vi "CODCr流程质控自动启动.vi"(0 "参数":T1={"是否启用仪器"=FALSE, "CODCr"={"启动测量模式"={"测量模式"=enum."水样测量"}, "确定按钮"=TRUE}, "启动模块"={"氨氮"=FALSE, "总磷"=FALSE, "总氮"=FALSE, "COD"=FALSE}, "常规启动"=FALSE, "直接启动"=FALSE}, 1 "CODCr量程切换":enum32{"H", "L", "AUTO"}(ring)=enum."AUTO" caption="CODMn量程切换") -> ()   [LabVIEW 2016, in "质控单元.lvlib"]
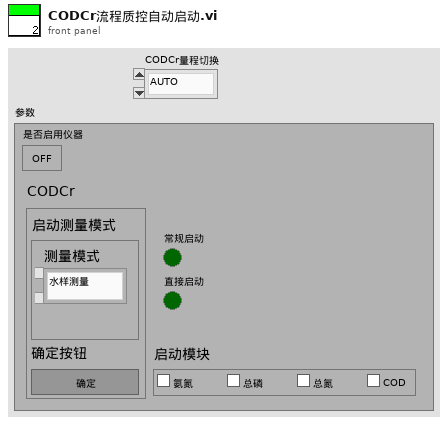
[diagram p1: front panel]
types:
  T1 = cluster{"是否启用仪器":bool, "CODCr":cluster{"启动测量模式":cluster{"测量模式":enum16{"水样测量", "标样核查", "加标回收", "平行样", "校零", "校标"}}, "确定按钮":bool}, "启动模块":cluster{"氨氮":bool, "总磷":bool, "总氮":bool, "COD":bool}, "常规启动":bool, "直接启动":bool}
  T2 = cluster{"R0":i16, "R1":i16, "R2":i16, "R3":i16, "R4":i16, "R5":i16, "R6":i16, "R7":i16, "R8":i16, "R9":i16, "R10":i16, "R11":i16, "R12":i16, "R13":i16, "R14":i16, "R15":i16, "R16":i16, "R17":i16, "R18":i16, "R19":i16, "R20":i16, "R21":i16, "R22":i16, "R23":i16, "R24":i16, "R25":i16, "R26":i16, "R27":i16, "R28":i16, "R29":i16, "R30":i16, "R31":i16, "R32":i16, "R33":i16, "R34":i16, "R35":i16, "R36":i16, "R37":i16, "R38":i16, "R39":i16, "R40":i16, "R41":i16, "R42":i16, "R43":i16, "R44":i16, "R45":i16, "R46":i16, "R47":i16, "R48":i16, "R49":i16, "R50":i16, "R51":i16, "R52":i16, "R53":i16, "R54":i16, "R55":i16, "R56":i16}
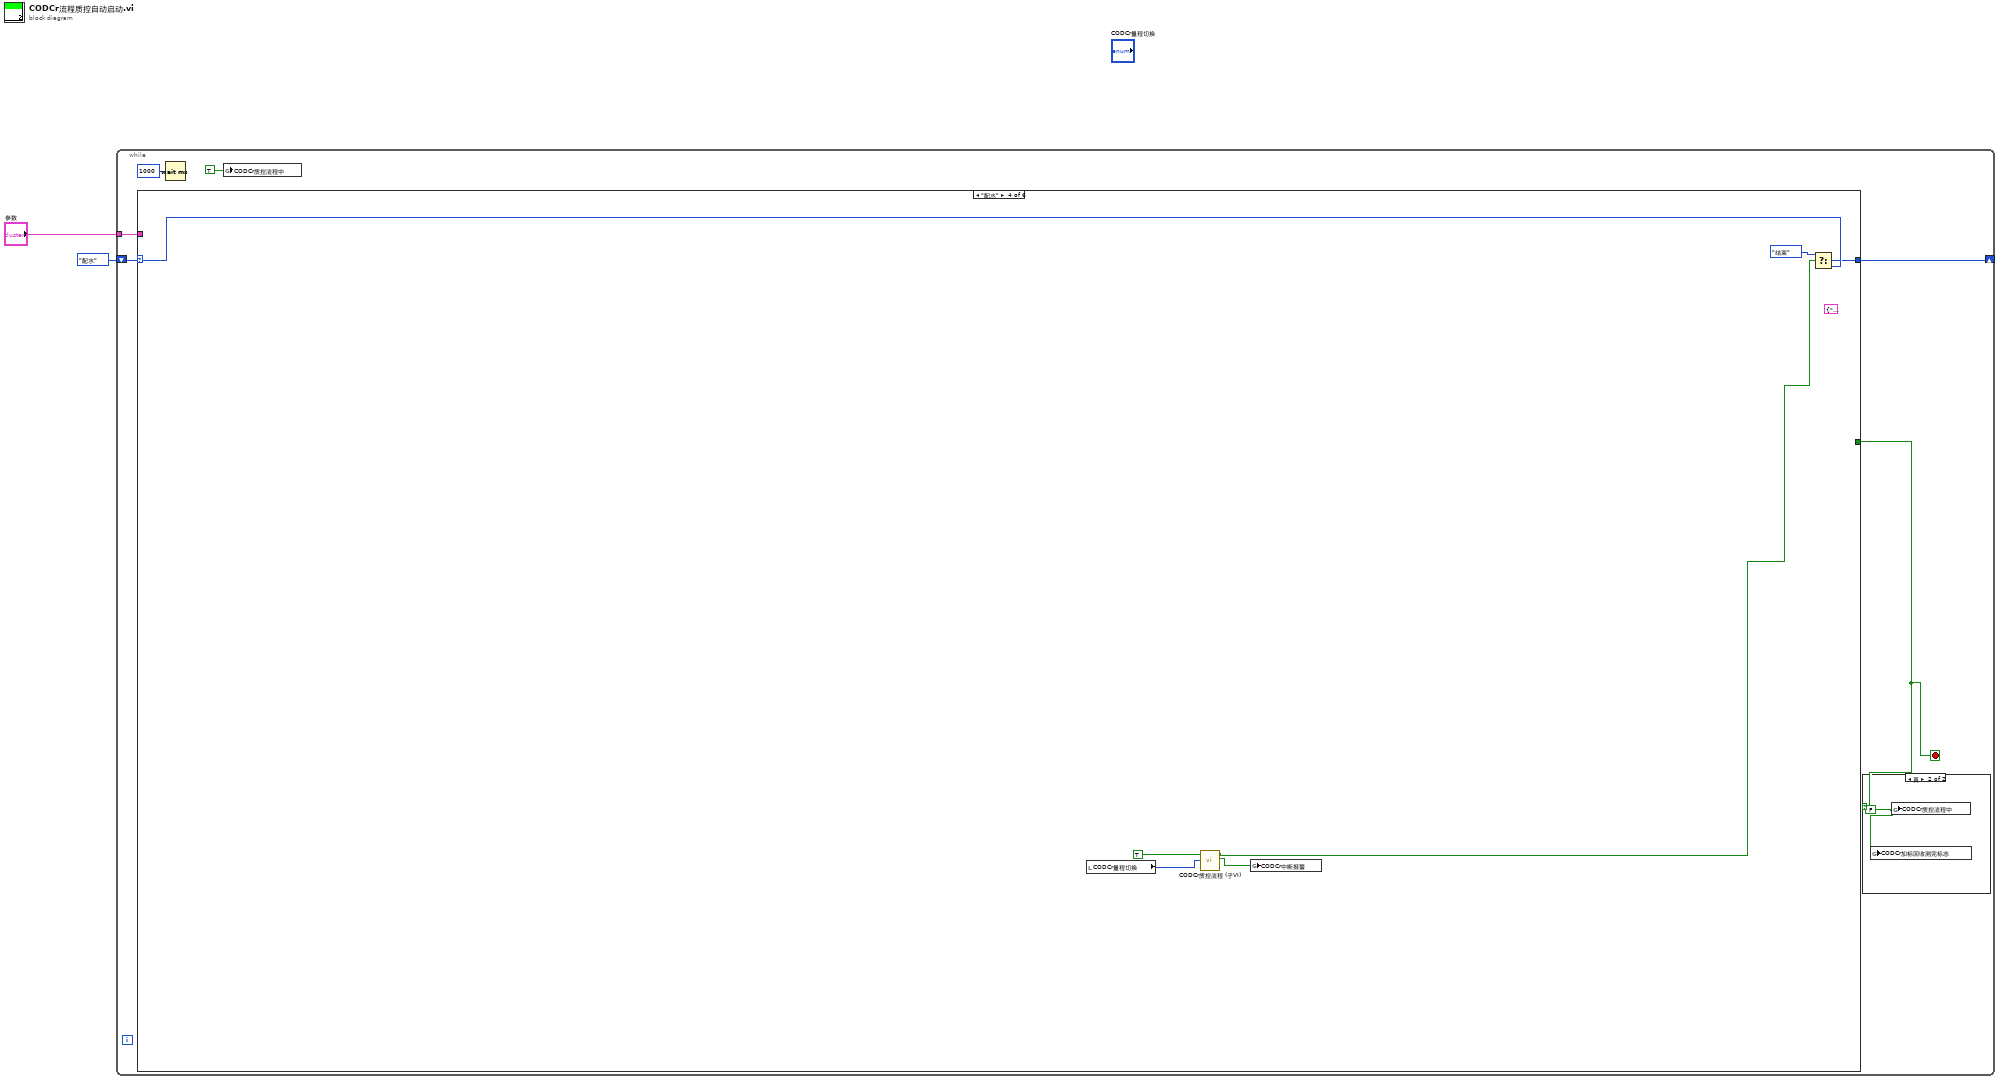
[diagram p0: block diagram]
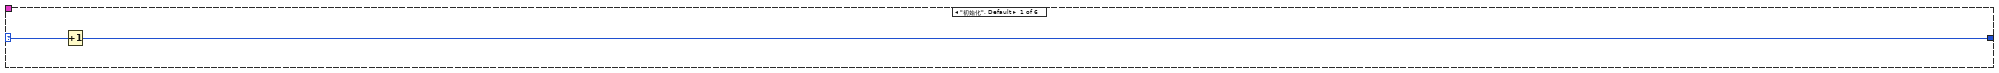
[diagram p3: hidden frame]
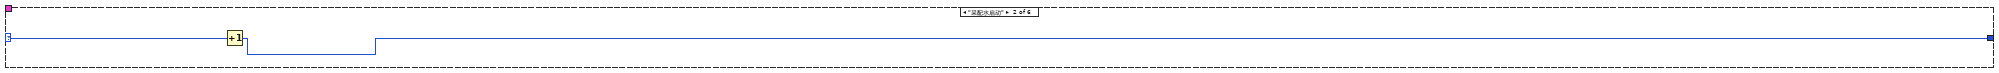
[diagram p4: hidden frame]
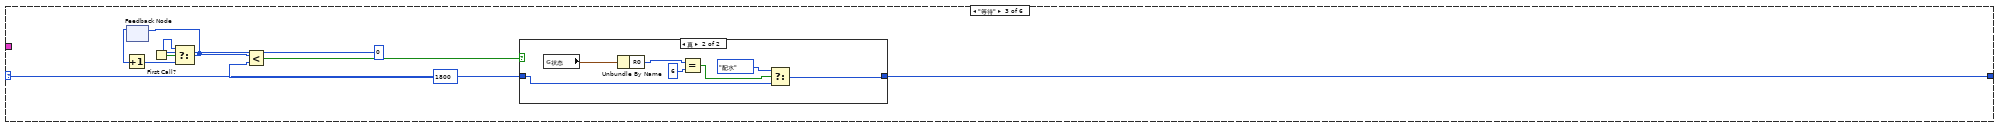
[diagram p5: hidden frame]
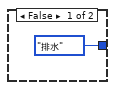
[diagram p6: hidden frame]
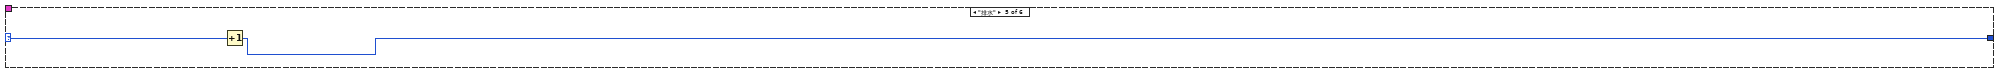
[diagram p7: hidden frame]
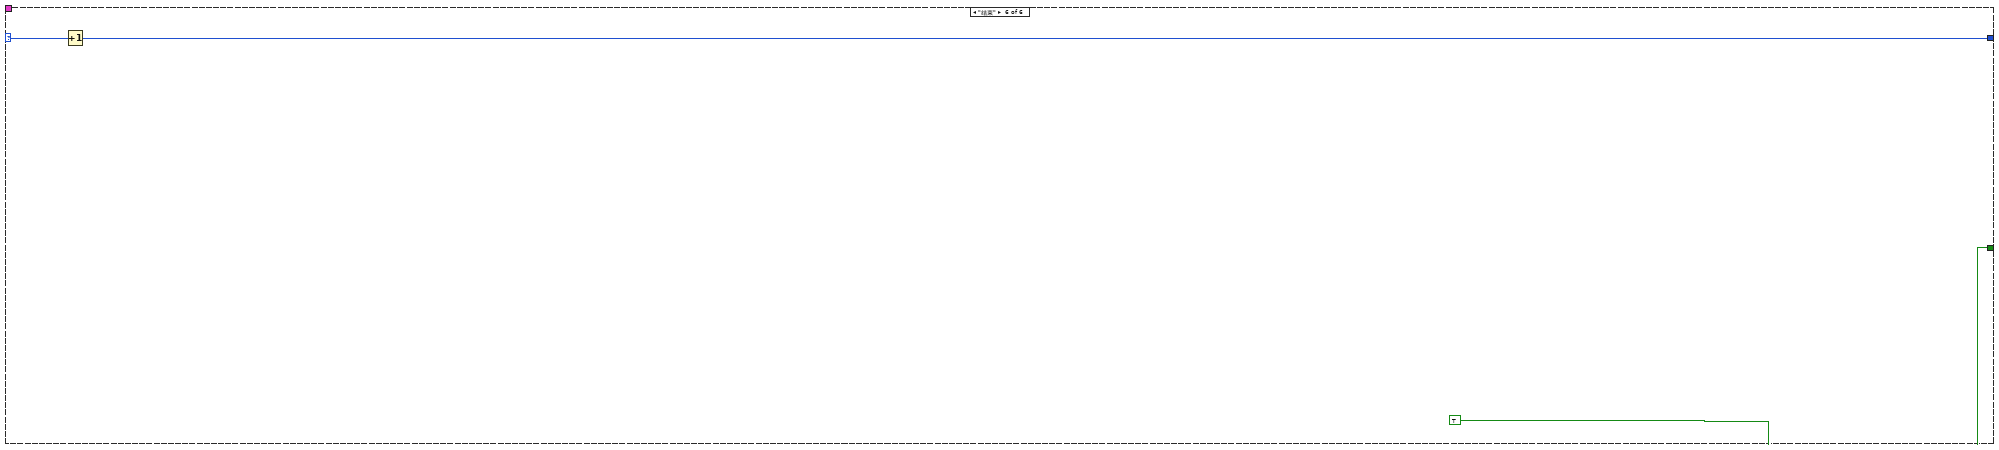
[diagram p8: hidden frame]
diagram:
  n1 = while {
    shift-right: [w7] -> _
    shift-left: enum16{"初始化", "采配水启动", "等待", "配水", "排水", "结束"}."配水" ("枚举") -> [w8]
    tunnel: "参数" -> [w5]
    stop <- w3 stop-if-true
    n2 = case shown="\"配水\"" w8 {
      selector: w8 -> [w11 w13 w20 w36 w39 w42]
      tunnel: [w10 w12 w19 w35 w38 w41] -> w7
      tunnel: [_ _ _ _ _ TRUE] -> w3
      tunnel: w5 -> [_ _ _ _ _ _]
      frame "初始化", Default {
        n3 = Increment(x=w11) -> (x+1=w10:enum16{"初始化", "采配水启动", "等待", "配水", "排水", "结束"})
      }
      frame "采配水启动" {
        n4 = Increment(x=w13) -> (x+1=w12:enum16{"初始化", "采配水启动", "等待", "配水", "排水", "结束"})
      }
      frame "等待" {
        n5 = feedback #1() -> (w16:i32)  [unwired: 1 in]
        n6 = Increment(x=w16) -> (x+1=w15:i32)
        n7 = First Call?() -> (First Call?: T/F=w17:bool)
        n8 = Select(t=0, s=w17, f=w15) -> (s? t:f=w14:i32)
        n9 = feedback-in #1(w14) -> ()
        n10 = Less?(x=w14, y=1800) -> (x < y?=w21:bool)
        n11 = case shown="真" w21 {
          tunnel: w20 -> [_ w26]
          tunnel: [enum16{"初始化", "采配水启动", "等待", "配水", "排水", "结束"}."排水" ("枚举") w25] -> w19
          frame False {
          }
          frame True {
            n12 = global read "与采配水交互全局.vi" "状态"() -> (w24:T2)
            n13 = Unbundle By Name(w24) -> ("R0"=w30:i16)
            n14 = Equal?(x=w30, y=i16 6) -> (x = y?=w28:bool)
            n15 = Select(t=enum16{"初始化", "采配水启动", "等待", "配水", "排水", "结束"}."配水" ("枚举"), s=w28, f=w26) -> (s? t:f=w25:enum16{"初始化", "采配水启动", "等待", "配水", "排水", "结束"})
          }
        }
      }
      frame "配水" {
        (unwired) cluster{"命令":string, "data":variant} {"命令"="启动", "data"=variant(cluster{"站号":u16, "控制命令输出":u16[]} {"站号"=1, "控制命令输出"=[256, 0]})} ("元素")
        n16 = local read "CODCr量程切换"() -> (w33:enum32{"H", "L", "AUTO"})
        n17 = call "CODCr质控流程 (子VI).vi"("CODCr量程切换"=w33, "CODCr"=TRUE) -> ("CODCr中断报警"=w31:bool, "布尔"=w32:bool)  [unwired: 8 in]
        n18 = global write "质控中断报警全局.vi" "CODCr中断报警"(w31) -> ()
        n19 = Select(t=enum16{"初始化", "采配水启动", "等待", "配水", "排水", "结束"}."结束" ("枚举"), s=w32, f=w36) -> (s? t:f=w35:enum16{"初始化", "采配水启动", "等待", "配水", "排水", "结束"})
      }
      frame "排水" {
        n20 = Increment(x=w39) -> (x+1=w38:enum16{"初始化", "采配水启动", "等待", "配水", "排水", "结束"})
      }
      frame "结束" {
        n21 = Increment(x=w42) -> (x+1=w41:enum16{"初始化", "采配水启动", "等待", "配水", "排水", "结束"})
      }
    }
    n22 = Wait (ms)(milliseconds to wait=u32 1000 ("等待时间（毫秒）")) -> ()  [unwired: 1 out]
    n23 = global write "质控测完标志全局 1.vi" "CODCr质控流程中"(TRUE ("氨氮质控流程中")) -> ()
    n24 = case shown="真" w3 {
      frame False {
      }
      frame True {
        w9 = FALSE ("氨氮质控流程中")
        n25 = global write "质控测完标志全局 1.vi" "CODCr加标回收测完标志"(w9) -> ()
        n26 = global write "质控测完标志全局 1.vi" "CODCr质控流程中"(w9) -> ()
      }
    }
  }
